vi "FTW-Connector-SendPoisonPill.vi"(0 "FTW Actor Connector":T1, 5 "Timeout":i32=1000 format="%dmsec", 11 "error in":errorcluster) -> (4 "FTW Actor Connector out":T1, 6 "Shutting Down?":bool, 8 "Roundtrip Time":dbl format="%.4psec", 15 "error out":errorcluster)   [LabVIEW 2015]
uses:
  core/type/FTW-Type-Actor-Connector.ctl
  time/FTW-Time-RelativeTimer.vi
  error/FTW-ERR-ThrowError.vi
  reflection/FTW-Reflection-Type.vi
  error/FTW-ERR-CallChain.vi
  string/FTW-STR-ReplaceWhitespace.vi
  reflection/FTW-Reflection-Array.vi
  string/FTW-STR-Array-Delimit.vi
  lib/FTW-KernelFilepath.vi
  json/core/FTW-JSON-Core-EncodingFlags.vi
  codegen/xnode/json/fetch/FTW-JSON-Core-GetFlattenedValue.vi
  support/FTW-Socket-Core-LibraryError.vi
  actor/request/FTW-Request-InterpretResponse.vi
  codegen/xnode/FTW-Actor-Ask.xnode
  codegen/xnode/FTW-JSON-Fetch.xnode
panel:
  # "Inputs"
  # "Outputs"
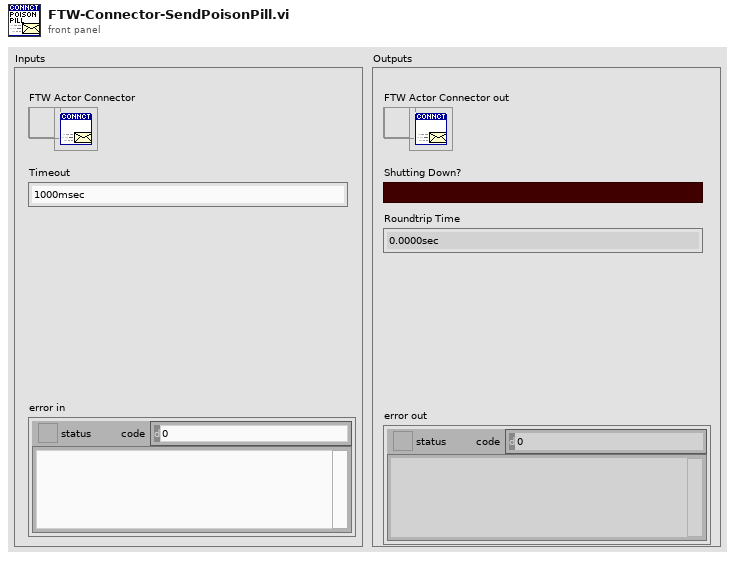
[diagram p1: front panel]
types:
  T1 = typedef "FTW-Type-Actor-Connector.ctl" = refnum<data-value>
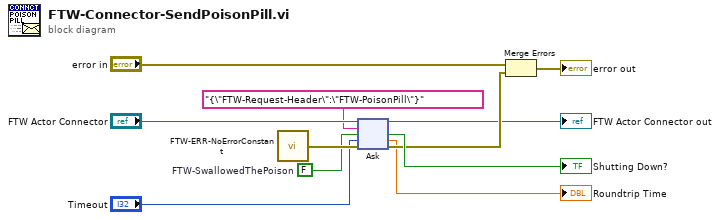
[diagram p0: block diagram]
diagram:
  w2 = FALSE  # FTW-SwallowedThePoison
  n1 = call "FTW-ERR-NoErrorConstant.vi"() -> ("no error"=w8:errorcluster)
  n2 = xnode "Ask"("FTW Actor Connector"="FTW Actor Connector", "Request"="{\"FTW-Request-Header\":\"FTW-PoisonPill\"}", "Response Type and Defaults"=w2, "Timeout"="Timeout", "error in"=w8) -> ("FTW Actor Connector out"=→"FTW Actor Connector out":T1, "Response"=→"Shutting Down?":bool, "Roundtrip Time"=→"Roundtrip Time":dbl, "error out"=w5:errorcluster)
  n3 = Merge Errors("error in", w5) -> (→"error out":errorcluster)
